vi "Read Data.vi"(8 "error in (no error)":errorcluster, 11 "LR-700 in":refnum<class "LR-700.lvclass">) -> (0 "error out":errorcluster, 2 "Data":waveform(dbl)[](array[waveform]), 3 "LR-700 out":refnum<class "LR-700.lvclass">)   [LabVIEW 2015, in "LR-700.lvclass"]
uses:
  LR-700.lvclass
  Instrument with scanner/Instrument with scanner Front Panel Data.ctl
  OO Devices/Device/Read Controls Snapshot.vi
  Instrument/Read VISA Resource.vi
  OO Devices/Device/Read Control Panel Loaded.vi
  Instrument/Write VISA Resource.vi
  Instrument with scanner/Instrument with scanner.lvclass
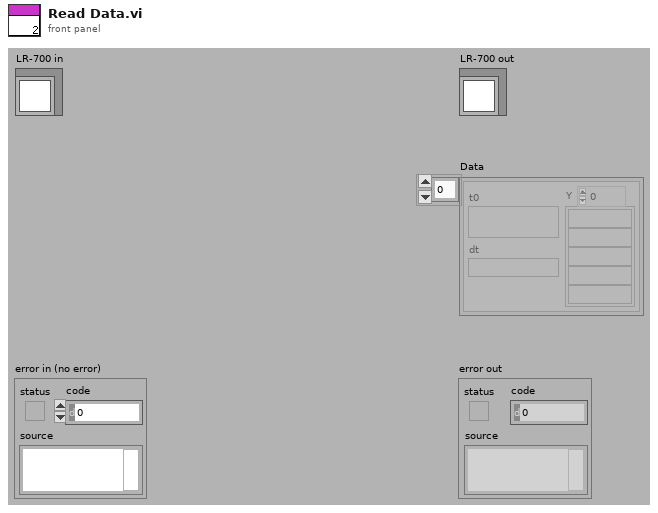
[diagram p1: front panel]
types:
  T1 = typedef "Instrument with scanner Front Panel Data.ctl" = cluster{"Channels to scan":i32[], "Scan settling, s":dbl}
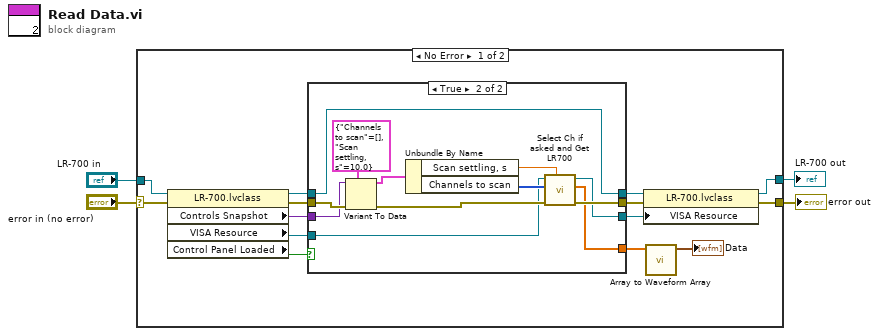
[diagram p0: block diagram]
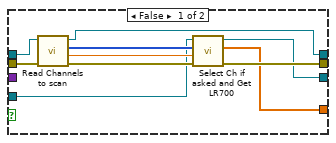
[diagram p2: hidden frame]
diagram:
  n1 = case shown="No Error" "error in (no error)" {
    selector: "error in (no error)" -> [w17 w42]
    tunnel: [w15 w42] -> w3
    tunnel: [w16 w41] -> w1
    tunnel: "LR-700 in" -> [w18 w41]
    frame No Error {
      n2 = property class="LR-700.lvclass"(reference=w18, error in=w17) -> (reference out=w9:refnum<class "LR-700.lvclass">, error out=w12:errorcluster, "Controls Snapshot"=w5:variant, "VISA Resource"=w7:refnum<visa-resource-name>, "Control Panel Loaded"=w6:bool)
      n3 = case shown="True" w6 {
        tunnel: [w28 w32] -> w14
        tunnel: [w27 w33] -> w13
        tunnel: w12 -> [w25 w40]
        tunnel: [w22 w29] -> w10
        tunnel: w9 -> [w21 w32]
        tunnel: [w20 w30] -> w8
        tunnel: w7 -> [w19 w31]
        tunnel: w5 -> [_ w39]
        frame False {
          n4 = call "Read Channels to scan.vi"("error in (no error)"=w25, "Instrument with scanner.lvclass in"=w21) -> ("error out"=w26:errorcluster, "Seconds between samples"=w23:dbl, "Channels to scan (empty - don't use scanner option)"=w24:i32[], "Instrument with scanner.lvclass out"=w28:refnum<class "LR-700.lvclass">)  [unwired: 6 out]
          n5 = call "Select Ch if asked and Get LR700.vi"("Seconds between samples"=w23, "error in (no error)"=w26, "Channels to scan (empty - don't use scanner option)"=w24, "VISA Resource Name"=w19) -> ("error out"=w27:errorcluster, "Data"=w22:dbl[], "VISA resource name out"=w20:refnum<visa-resource-name>)  [unwired: 5 out]
        }
        frame True {
          n6 = Variant To Data(error in=w40, type=T1 {"Channels to scan"=[], "Scan settling, s"=10.0} ("Data"), Variant=w39) -> (data=w37:T1, error out=w36:errorcluster)
          n7 = Unbundle By Name(w37) -> ("Scan settling, s"=w35:dbl, "Channels to scan"=w34:i32[])
          n8 = call "Select Ch if asked and Get LR700.vi"("Seconds between samples"=w35, "error in (no error)"=w36, "Channels to scan (empty - don't use scanner option)"=w34, "VISA Resource Name"=w31) -> ("error out"=w33:errorcluster, "Data"=w29:dbl[], "VISA resource name out"=w30:refnum<visa-resource-name>)  [unwired: 5 out]
        }
      }
      n9 = property class="LR-700.lvclass"(reference=w14, error in=w13, "VISA Resource"=w8) -> (reference out=w16:refnum<class "LR-700.lvclass">, error out=w15:errorcluster)
      n10 = call "Array to Waveform Array.vi"("Array"=w10) -> ("Waveform"=→"Data":waveform(dbl)[])  [unwired: 10 in]
    }
    frame Error {
    }
  }
  "error out" <- w3
  "LR-700 out" <- w1
